vi "get conex position from DB.vi"(8 "error in (no error)":errorcluster, 11 "Device/Devicetype name\n/Plotter.id/ScanName#":string) -> (0 "error out":errorcluster, 3 "postiionn from DB":string)   [LabVIEW 2020]
uses:
  Shared/MySQL/Preset Query Enum.ctl
panel:
  out "data":string[][](array[string])
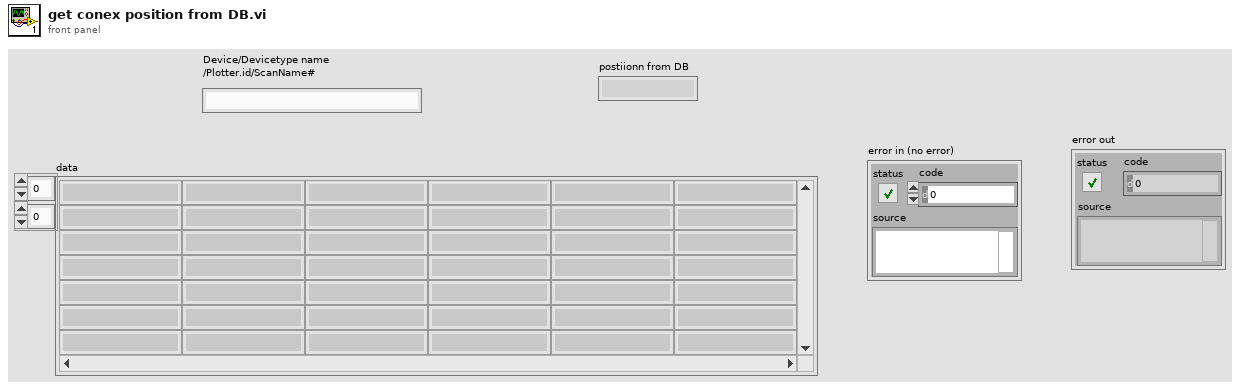
[diagram p1: front panel]
types:
  T1 = typedef "Preset Query Enum.ctl" = enum16{"Get Locations", "Get all IPs and MACs", "Get classes", "Get expt variables to set at scanstart for particular device", "Get expt devices and variables with start values", "Get expt devices and variables (with data to get)", "Get expt devices with data to get", "Get Expt devices and GUIs", "Get all devices basic properties", "Get Virtual Devices Core Info", "Get Expt names", "Get experiment basic properties", "Get experiment alarm variables", "Get MC Ports", "Get device network comm port", "Get devicetype lvclass path", "Get basic device properties", "Get Init Order", "Get all setable variables of a device", "Get device variable aliases", "Get force values of all settable variables", "Get all variables of a devicetype", "Get all variables of a device", "Get plotter details", "Get Saved Scans", "Get Scan Info", "GetGeneralGUIs", "Get expt for plotter", "Get plotter IDs from expt", "Get all devices", "Get all Virtual Devices", "Get all aliases", "Get variable and device info for Virtual Device", "GetItemLocatorIP", "Get IPs for GUIs", "Get DeviceType from Device", "GetLocalPortRange", "GetDevicePresetVariables", "Get Device Configuration", "GetAllPresetNames", "GetAllConfigurationNames", "GetPresetDeviceNames", "GetDeviceAliases", "GetDevicesOfClass"}
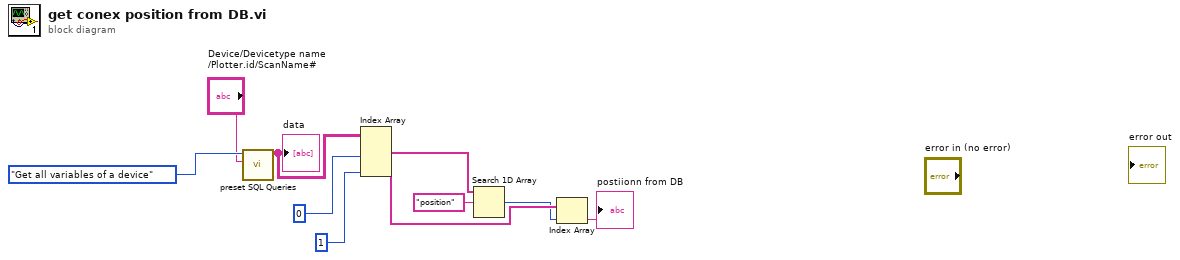
[diagram p0: block diagram]
diagram:
  n1 = call "preset SQL Queries.vi"("Device/Devicetype name\n/Plotter.id/ScanName#"="Device/Devicetype name\n/Plotter.id/ScanName#", "Preset Query"=Preset_Query_Enum."Get all variables of a device") -> ("data"=w8:string[][])  [unwired: 7 in, 2 out]
  "data" <- w8
  n2 = Index Array(array=w8, index (col) #1=0 ("disabled index (col)"), index (col) #2=1 ("index (col)")) -> (element #1=w5:string[], element #2=w3:string[])  [unwired: 2 in]
  n3 = Search 1D Array(1D array=w5, element="position") -> (index of element=w2:i32)  [unwired: 1 in]
  n4 = Index Array(array=w3, index=w2) -> (element=→"postiionn from DB":string)
